vi "CalculoDistanciaGeografica.vi"(2 "Current Location (degrees)":cluster{"Latitude":dbl, "Longitude":dbl} {"Longitude" format="%#.6g"; "Latitude" format="%#.6g"}, 3 "Destination (degrees)":cluster{"Latitude":dbl, "Longitude":dbl} {"Longitude" format="%#.6g"; "Latitude" format="%#.6g"}) -> (0 "Distance to Destination m":dbl, 1 "Distance to Destination km":dbl)   [LabVIEW 2017]
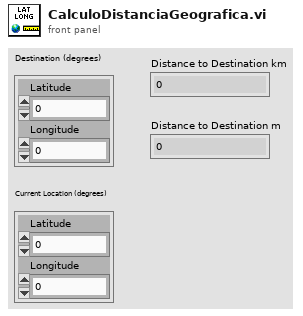
[diagram p1: front panel]
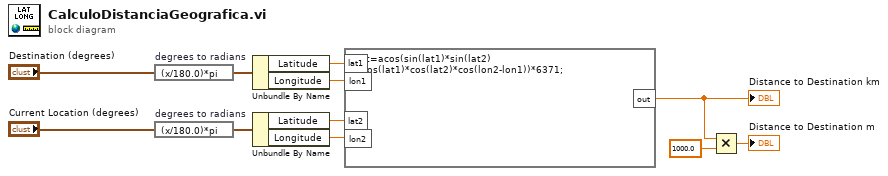
[diagram p0: block diagram]
diagram:
  n1 = expression code="(x/180.0)*pi" "degrees to radians"("Destination (degrees)") -> (w3:cluster{"Latitude":dbl, "Longitude":dbl})
  n2 = expression code="(x/180.0)*pi" "degrees to radians"("Current Location (degrees)") -> (w2:cluster{"Latitude":dbl, "Longitude":dbl})
  n3 = Unbundle By Name(w3) -> ("Latitude"=w9:dbl, "Longitude"=w8:dbl)
  n4 = Unbundle By Name(w2) -> ("Latitude"=w11:dbl, "Longitude"=w10:dbl)
  n5 = formula code="out=acos(sin(lat1)*sin(lat2)\n+cos(lat1)*cos(lat2)*cos(lon2-lon1))*6371;"("lat1"=w9, "lat2"=w11, "lon1"=w8, "lon2"=w10) -> ("out"=w7:dbl)
  "Distance to Destination km" <- w7
  n6 = Multiply(x=w7, y=1000.0) -> (x*y=→"Distance to Destination m":dbl)
